vi "rqc Clock Generator.vi"(2 "reset":bool, 5 "SCTL clock devider":u8=2 min=2 step=1) -> (6 "clock out":bool)   [LabVIEW 2018]
doc: "Generates clock signal. Should be placed in SCTL.\n<b>cock out</b> frequency = SCTL clock frequency /(2^ <b>SCTL clock devider</b>)\n<b>SCTL clock devider</b> shold be greater or equal to 1."
uses:
  <vilib>/RQC/FPGA Basic Logic/Counters/Counter (U8).vi
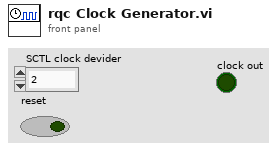
[diagram p1: front panel]
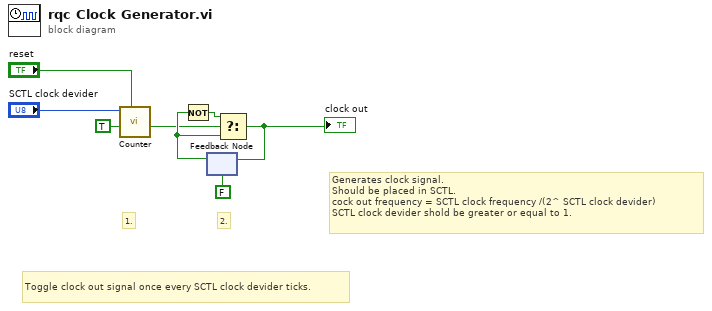
[diagram p0: block diagram]
diagram:
  # "Toggle clock out signal once every SCTL clock devider ticks."
  # "2."
  # "1."
  # "Generates clock signal. \nShould be placed in SCTL.\ncock out frequency = SCTL clock frequency /(2^ SCTL clock devider)\nSCTL clock devider shold be greater or equal to 1."
  n1 = call-poly <vilib>:"Counter.vi"("reset"="reset", "increment"=TRUE, "bound"="SCTL clock devider") -> ("done"=w5:bool)  [unwired: 7 in, 1 out]
  n2 = feedback #1(FALSE) -> (w6:bool)
  n3 = Not(x=w6) -> (.not. x?=w7:bool)
  n4 = Select(t=w7, s=w5, f=w6) -> (s? t:f=w4:bool)
  "clock out" <- w4
  n5 = feedback-in #1(w4) -> ()
